vi "serial_connect.vi"(7 "button_serial_connect":bool, 8 "error_in":errorcluster, 9 "serial_connected_in":bool, 11 "VISA_resource":refnum<visa-resource-name>) -> (0 "error out":errorcluster, 1 "serial_connected_out":bool, 2 "new_connection":bool, 3 "VISA_refnum_out":refnum<visa-resource-name>)   [LabVIEW 2025]
uses:
  <vilib>/Instr/_visa.llb/VISA Configure Serial Port (Instr).vi
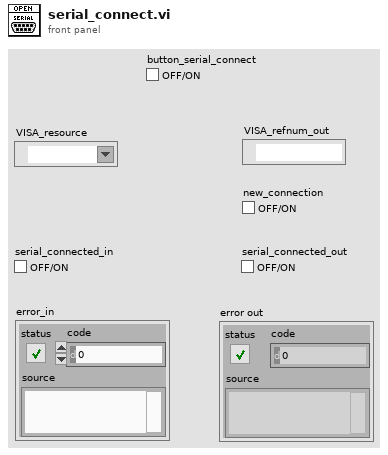
[diagram p1: front panel]
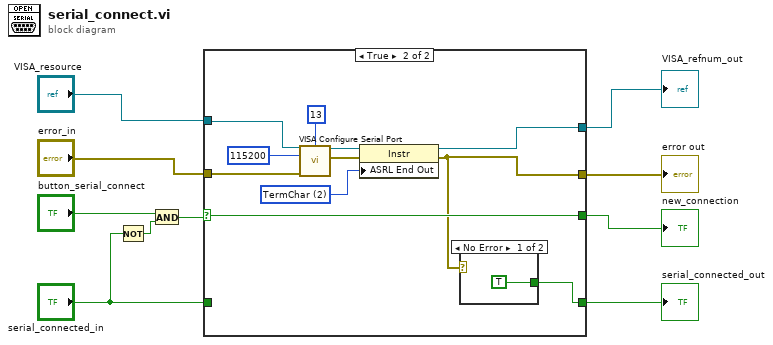
[diagram p0: block diagram]
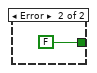
[diagram p3: hidden frame]
diagram:
  n1 = Not(x="serial_connected_in") -> (.not. x?=w3:bool)
  n2 = And(x="button_serial_connect", y=w3) -> (x .and. y?=w5:bool)
  n3 = case shown="True" w5 {
    selector: w5 -> [w12 w17]
    tunnel: [w13 w19] -> w8
    tunnel: [_ w16] -> w9
    tunnel: "VISA_resource" -> [w13 w18]
    tunnel: [w12 w17] -> w7
    tunnel: [w11 w15] -> w6
    tunnel: "serial_connected_in" -> [w11 _]
    tunnel: "error_in" -> [_ w14]
    frame False {
    }
    frame True {
      w22 = u16 2 items=["None", "Last Bit", "TermChar", "Break"] ("Serial Settings:End Mode for Writes")
      n4 = call-poly "VISA Configure Serial Port"("VISA resource name"=w18, "termination char\n(0xA = '\\n' = LF)"=u8 13 ("termination char\n(0xA = '\\n' = LF)"), "baud rate (9600)"=u32 115200, "error in (no error)"=w14) -> ("VISA resource name out"=w23:refnum<visa-resource-name>, "error out"=w24:errorcluster)  [unwired: 10 in]
      n5 = property class="Instr"(reference=w23, error in=w24, "ASRL End Out"=w22) -> (reference out=w19:refnum<visa-resource-name>, error out=w16:errorcluster)
      n6 = case shown="No Error" w16 {
        tunnel: [TRUE ("serial_connected_in") FALSE ("serial_connected_in")] -> w15
        frame No Error {
        }
        frame Error {
        }
      }
    }
  }
  "error out" <- w9
  "VISA_refnum_out" <- w8
  "new_connection" <- w7
  "serial_connected_out" <- w6
